vi "Check Config.vi"(8 "error in (no error)":errorcluster) -> (0 "error out":errorcluster, 3 "Config Check Results":T1[](array[typedef]))   [LabVIEW 2026, in "Readines Service.lvclass"]
uses:
  Readines Service.lvclass
  Readines Service.lvclass/Readines Service.ctl
  Typedefs/enums/Readiness State Enum.ctl
  Typedefs/clusters/Readiness Check Result.ctl
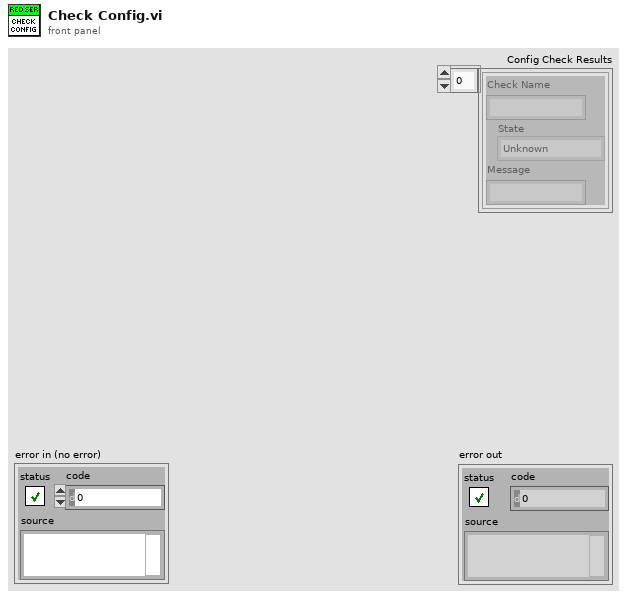
[diagram p1: front panel]
types:
  T1 = typedef "Readiness Check Result.ctl" = cluster{"Check Name":string, "State":T2, "Message":string}
  T2 = typedef "Readiness State Enum.ctl" = enum16{"Unknown", "Ready", "Warning", "NotReady"}
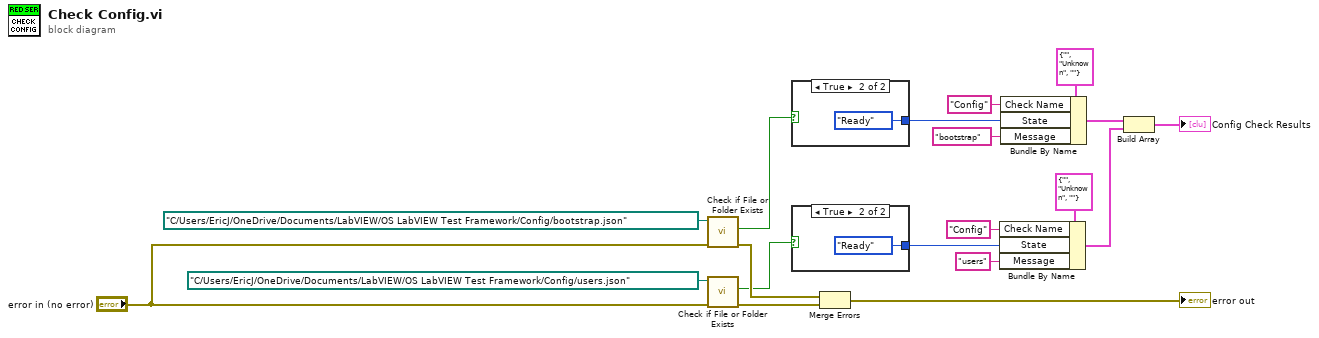
[diagram p0: block diagram]
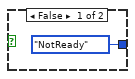
[diagram p2: hidden frame]
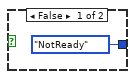
[diagram p3: hidden frame]
diagram:
  n1 = call <vilib>:"Check if File or Folder Exists.vi"("error in (no error)"="error in (no error)", "path"=path "C:/Users/EricJ/OneDrive/Documents/LabVIEW/OS LabVIEW Test Framework/Config/bootstrap.json") -> ("error out"=w16:errorcluster, "file or folder exists?"=w11:bool)  [unwired: 7 in, 1 out]
  n2 = call <vilib>:"Check if File or Folder Exists.vi"("error in (no error)"="error in (no error)", "path"=path "C:/Users/EricJ/OneDrive/Documents/LabVIEW/OS LabVIEW Test Framework/Config/users.json") -> ("error out"=w15:errorcluster, "file or folder exists?"=w5:bool)  [unwired: 7 in, 1 out]
  n3 = case shown="True" w11 {
    tunnel: [Readiness_State_Enum."NotReady" ("State") Readiness_State_Enum."Ready" ("State")] -> w10
    frame False {
    }
    frame True {
    }
  }
  n4 = case shown="True" w5 {
    tunnel: [Readiness_State_Enum."NotReady" ("State") Readiness_State_Enum."Ready" ("State")] -> w4
    frame False {
    }
    frame True {
    }
  }
  n5 = Merge Errors(w16, w15) -> (→"error out":errorcluster)
  n6 = Bundle By Name(cluster=T1 {"Check Name"="", "State"=enum."Unknown", "Message"=""} ("Readiness Check Result"), "Check Name"="Config", "State"=w4, "Message"="users") -> (w2:T1)
  n7 = Bundle By Name(cluster=T1 {"Check Name"="", "State"=enum."Unknown", "Message"=""} ("Readiness Check Result"), "Check Name"="Config", "State"=w10, "Message"="bootstrap") -> (w3:T1)
  n8 = Build Array(w3, w2) -> (→"Config Check Results":T1[])
